vi "Untitled 1 (SubVI).vi"(11 "Path":path) -> (3 "new picture":picture)   [LabVIEW 2020]
panel:
  # "Ceballos Conde Emanuel"
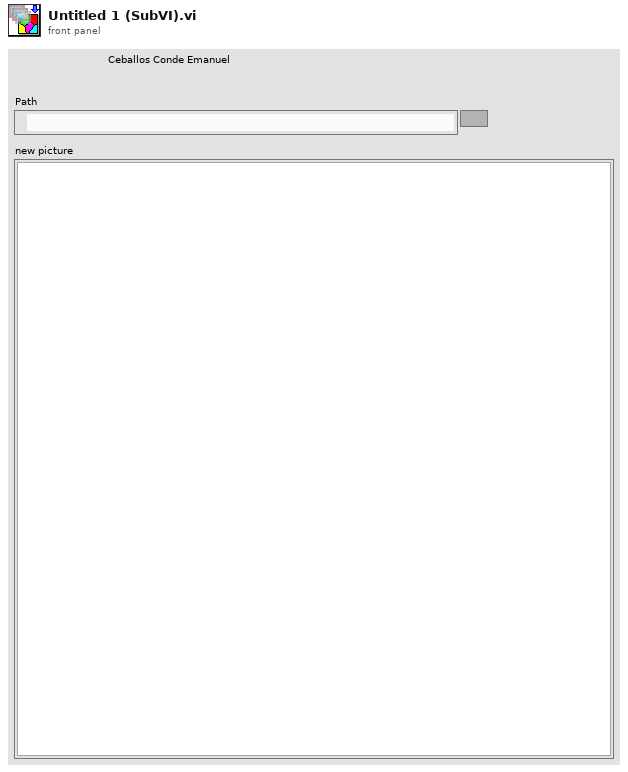
[diagram p1: front panel]
types:
  T1 = enum16{"E1", "E2", "E3", "E4", "E5", "E6", "E7", "E8", "E9"}
  T2 = typedef "imagedata.ctl" = cluster{"image type":i32, "image depth":i32, "image":u8[], "mask":u8[], "colors":u32[], "Rectangle":cluster{"left":i16, "top":i16, "right":i16, "bottom":i16}}
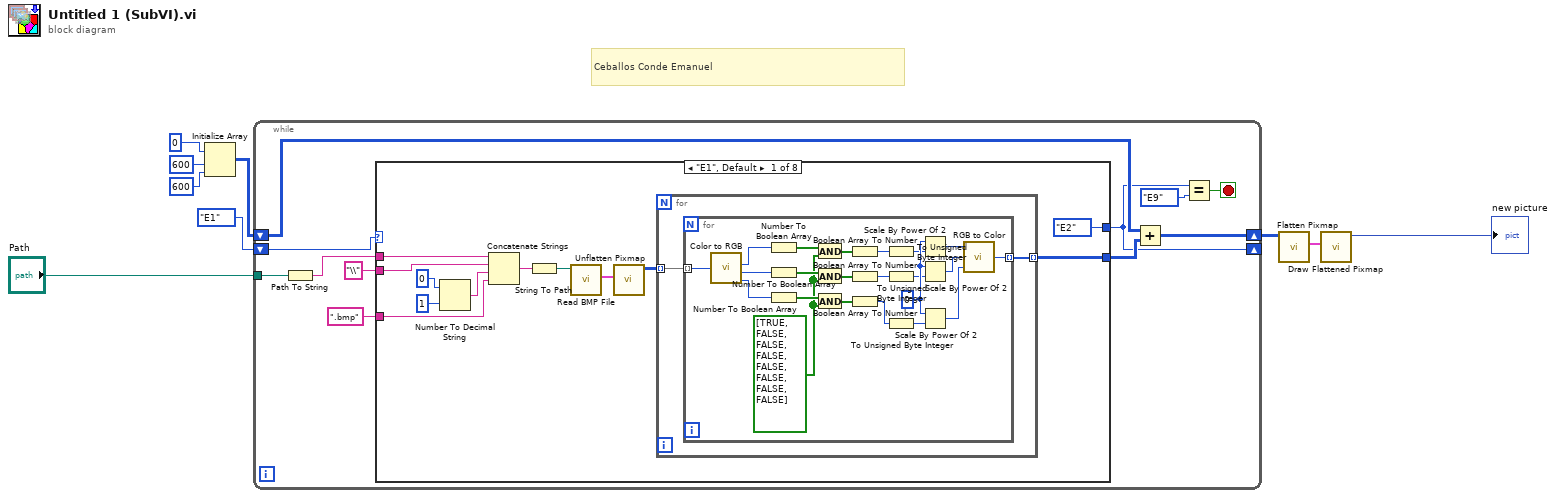
[diagram p0: block diagram]
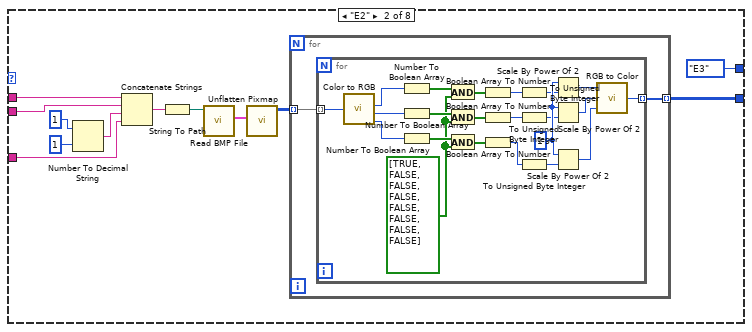
[diagram p2: hidden frame]
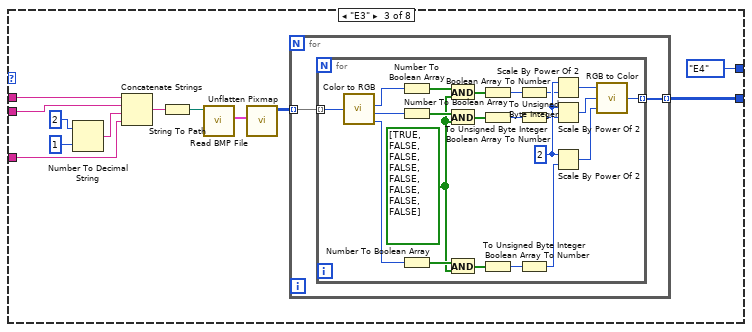
[diagram p3: hidden frame]
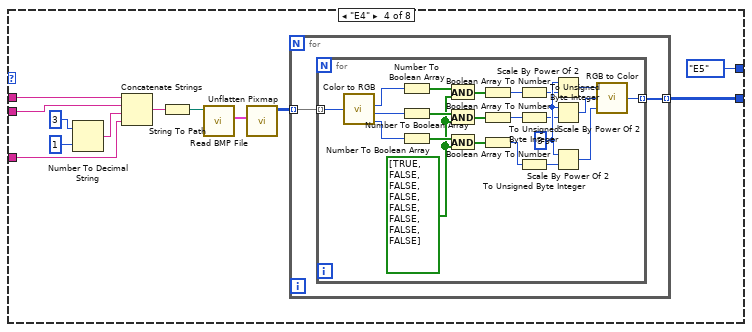
[diagram p4: hidden frame]
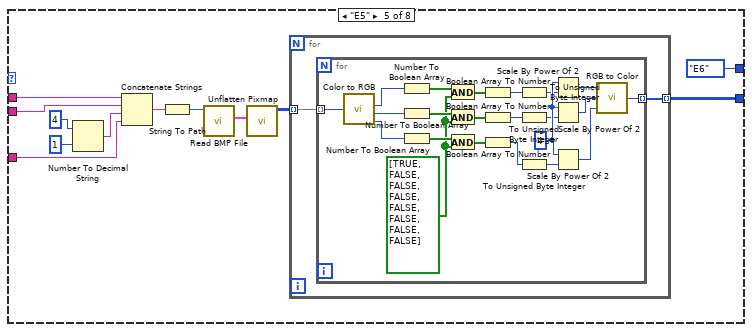
[diagram p5: hidden frame]
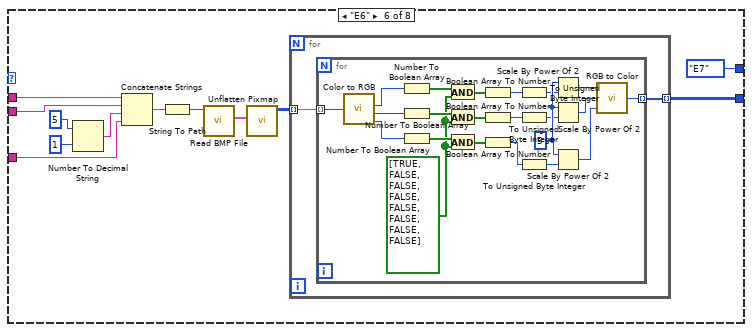
[diagram p6: hidden frame]
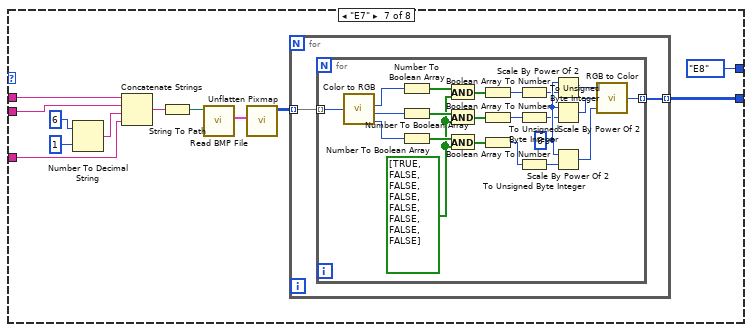
[diagram p7: hidden frame]
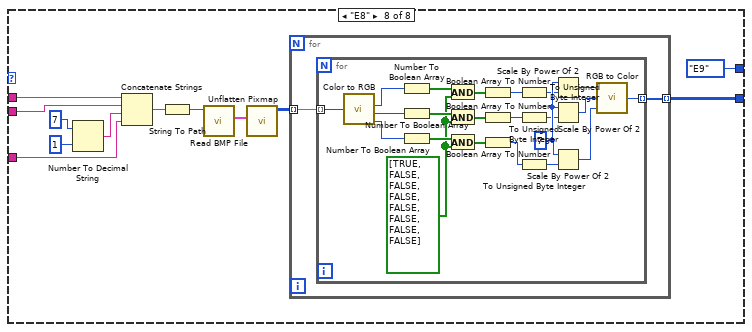
[diagram p8: hidden frame]
diagram:
  # "Ceballos Conde Emanuel"
  n1 = Initialize Array(u32 0 ("element"), 600 ("dimension size"), 600 ("dimension size")) -> (w5:u32[][])
  n2 = while {
    shift-right: [w15] -> _
    shift-left: T1."E1" -> [w20]
    shift-right: [w18] -> w4
    shift-left: w5 -> [w17]
    tunnel: "Path" -> [w10]
    stop <- w16 stop-if-true
    n3 = Path To String(path=w10) -> (string=w13:string)
    n4 = case shown="\"E1\", Default" w20 {
      tunnel: [w31 w66 w102 w138 w174 w210 w246 w282] -> w19
      tunnel: [T1."E2" T1."E3" T1."E4" T1."E5" T1."E6" T1."E7" T1."E8" T1."E9"] -> w15
      tunnel: w13 -> [w28 w60 w94 w130 w168 w205 w240 w276]
      tunnel: "\\" ("string") -> [w27 w59 w93 w129 w167 w204 w239 w275]
      tunnel: ".bmp" -> [w23 w57 w96 w132 w165 w203 w237 w273]
      frame "E1", Default {
        n5 = Number To Decimal String(number=0, width (-)=i16 1) -> (decimal integer string=w26:string)
        n6 = Concatenate Strings(w28, w27, w26, w23) -> (w21:string)
        n7 = String To Path(string=w21) -> (path=w22:path)
        n8 = call <vilib>:"Read BMP File.vi"("path to BMP file"=w22) -> ("image data"=w30:T2)  [unwired: 8 in, 2 out]
        n9 = call <vilib>:"Unflatten Pixmap.vi"("image data"=w30) -> ("24-bit pixmap"=w32:u32[][])  [unwired: 4 in, 6 out]
        n10 = for {
          tunnel: w32 -> [w34] mode=indexing
          tunnel: [w33] -> w31 mode=indexing
          n11 = for {
            tunnel: w34 -> [w56] mode=indexing
            tunnel: [w39] -> w33 mode=indexing
            w35 = bool[] [TRUE, FALSE, FALSE, FALSE, FALSE, FALSE, FALSE, FALSE] ("Boolean array 7")
            w42 = u8 0 ("x")
            n12 = call <vilib>:"Color to RGB.vi"("Color"=w56) -> ("R"=w53:u8, "G"=w48:u8, "B"=w47:u8)  [unwired: 1 out]
            n13 = Number To Boolean Array(number=w53) -> (Boolean array=w55:bool[])
            n14 = Number To Boolean Array(number=w48) -> (Boolean array=w52:bool[])
            n15 = Number To Boolean Array(number=w47) -> (Boolean array=w50:bool[])
            n16 = And(x=w55, y=w35) -> (x .and. y?=w54:bool[])
            n17 = And(x=w52, y=w35) -> (x .and. y?=w51:bool[])
            n18 = And(x=w50, y=w35) -> (x .and. y?=w49:bool[])
            n19 = Boolean Array To Number(Boolean array=w54) -> (number=w43:u32)
            n20 = Boolean Array To Number(Boolean array=w51) -> (number=w40:u32)
            n21 = Boolean Array To Number(Boolean array=w49) -> (number=w41:u32)
            n22 = To Unsigned Byte Integer(number=w43) -> (unsigned 8bit integer=w38:u8)
            n23 = To Unsigned Byte Integer(number=w40) -> (unsigned 8bit integer=w37:u8)
            n24 = To Unsigned Byte Integer(number=w41) -> (unsigned 8bit integer=w36:u8)
            n25 = Scale By Power Of 2(n=w42, x=w38) -> (x*2^n=w46:u8)
            n26 = Scale By Power Of 2(n=w42, x=w37) -> (x*2^n=w45:u8)
            n27 = Scale By Power Of 2(n=w42, x=w36) -> (x*2^n=w44:u8)
            n28 = call <vilib>:"RGB to Color.vi"("B"=w44, "G"=w45, "R"=w46) -> ("Color"=w39:u32)
          }
        }
      }
      frame "E2" {
        n29 = Number To Decimal String(number=1, width (-)=i16 1) -> (decimal integer string=w58:string)
        n30 = Concatenate Strings(w60, w59, w58, w57) -> (w64:string)
        n31 = String To Path(string=w64) -> (path=w61:path)
        n32 = call <vilib>:"Read BMP File.vi"("path to BMP file"=w61) -> ("image data"=w68:T2)  [unwired: 8 in, 2 out]
        n33 = call <vilib>:"Unflatten Pixmap.vi"("image data"=w68) -> ("24-bit pixmap"=w67:u32[][])  [unwired: 4 in, 6 out]
        n34 = for {
          tunnel: w67 -> [w70] mode=indexing
          tunnel: [w69] -> w66 mode=indexing
          n35 = for {
            tunnel: w70 -> [w92] mode=indexing
            tunnel: [w75] -> w69 mode=indexing
            w71 = bool[] [TRUE, FALSE, FALSE, FALSE, FALSE, FALSE, FALSE, FALSE] ("Boolean array 7")
            w78 = u8 1 ("x")
            n36 = call <vilib>:"Color to RGB.vi"("Color"=w92) -> ("R"=w89:u8, "G"=w84:u8, "B"=w83:u8)  [unwired: 1 out]
            n37 = Number To Boolean Array(number=w89) -> (Boolean array=w91:bool[])
            n38 = Number To Boolean Array(number=w84) -> (Boolean array=w88:bool[])
            n39 = Number To Boolean Array(number=w83) -> (Boolean array=w86:bool[])
            n40 = And(x=w91, y=w71) -> (x .and. y?=w90:bool[])
            n41 = And(x=w88, y=w71) -> (x .and. y?=w87:bool[])
            n42 = And(x=w86, y=w71) -> (x .and. y?=w85:bool[])
            n43 = Boolean Array To Number(Boolean array=w90) -> (number=w79:u32)
            n44 = Boolean Array To Number(Boolean array=w87) -> (number=w76:u32)
            n45 = Boolean Array To Number(Boolean array=w85) -> (number=w77:u32)
            n46 = To Unsigned Byte Integer(number=w79) -> (unsigned 8bit integer=w74:u8)
            n47 = To Unsigned Byte Integer(number=w76) -> (unsigned 8bit integer=w73:u8)
            n48 = To Unsigned Byte Integer(number=w77) -> (unsigned 8bit integer=w72:u8)
            n49 = Scale By Power Of 2(n=w78, x=w74) -> (x*2^n=w82:u8)
            n50 = Scale By Power Of 2(n=w78, x=w73) -> (x*2^n=w81:u8)
            n51 = Scale By Power Of 2(n=w78, x=w72) -> (x*2^n=w80:u8)
            n52 = call <vilib>:"RGB to Color.vi"("B"=w80, "G"=w81, "R"=w82) -> ("Color"=w75:u32)
          }
        }
      }
      frame "E3" {
        n53 = Number To Decimal String(number=2, width (-)=i16 1) -> (decimal integer string=w95:string)
        n54 = Concatenate Strings(w94, w93, w95, w96) -> (w100:string)
        n55 = String To Path(string=w100) -> (path=w97:path)
        n56 = call <vilib>:"Read BMP File.vi"("path to BMP file"=w97) -> ("image data"=w104:T2)  [unwired: 8 in, 2 out]
        n57 = call <vilib>:"Unflatten Pixmap.vi"("image data"=w104) -> ("24-bit pixmap"=w103:u32[][])  [unwired: 4 in, 6 out]
        n58 = for {
          tunnel: w103 -> [w106] mode=indexing
          tunnel: [w105] -> w102 mode=indexing
          n59 = for {
            tunnel: w106 -> [w128] mode=indexing
            tunnel: [w111] -> w105 mode=indexing
            w107 = bool[] [TRUE, FALSE, FALSE, FALSE, FALSE, FALSE, FALSE, FALSE] ("Boolean array 7")
            w114 = u8 2 ("x")
            n60 = call <vilib>:"Color to RGB.vi"("Color"=w128) -> ("R"=w125:u8, "G"=w120:u8, "B"=w119:u8)  [unwired: 1 out]
            n61 = Number To Boolean Array(number=w125) -> (Boolean array=w127:bool[])
            n62 = Number To Boolean Array(number=w120) -> (Boolean array=w124:bool[])
            n63 = Number To Boolean Array(number=w119) -> (Boolean array=w122:bool[])
            n64 = And(x=w127, y=w107) -> (x .and. y?=w126:bool[])
            n65 = And(x=w124, y=w107) -> (x .and. y?=w123:bool[])
            n66 = And(x=w122, y=w107) -> (x .and. y?=w121:bool[])
            n67 = Boolean Array To Number(Boolean array=w126) -> (number=w115:u32)
            n68 = Boolean Array To Number(Boolean array=w123) -> (number=w112:u32)
            n69 = Boolean Array To Number(Boolean array=w121) -> (number=w113:u32)
            n70 = To Unsigned Byte Integer(number=w115) -> (unsigned 8bit integer=w110:u8)
            n71 = To Unsigned Byte Integer(number=w112) -> (unsigned 8bit integer=w109:u8)
            n72 = To Unsigned Byte Integer(number=w113) -> (unsigned 8bit integer=w108:u8)
            n73 = Scale By Power Of 2(n=w114, x=w110) -> (x*2^n=w118:u8)
            n74 = Scale By Power Of 2(n=w114, x=w109) -> (x*2^n=w117:u8)
            n75 = Scale By Power Of 2(n=w114, x=w108) -> (x*2^n=w116:u8)
            n76 = call <vilib>:"RGB to Color.vi"("B"=w116, "G"=w117, "R"=w118) -> ("Color"=w111:u32)
          }
        }
      }
      frame "E4" {
        n77 = Number To Decimal String(number=3, width (-)=i16 1) -> (decimal integer string=w131:string)
        n78 = Concatenate Strings(w130, w129, w131, w132) -> (w136:string)
        n79 = String To Path(string=w136) -> (path=w133:path)
        n80 = call <vilib>:"Read BMP File.vi"("path to BMP file"=w133) -> ("image data"=w140:T2)  [unwired: 8 in, 2 out]
        n81 = call <vilib>:"Unflatten Pixmap.vi"("image data"=w140) -> ("24-bit pixmap"=w139:u32[][])  [unwired: 4 in, 6 out]
        n82 = for {
          tunnel: w139 -> [w142] mode=indexing
          tunnel: [w141] -> w138 mode=indexing
          n83 = for {
            tunnel: w142 -> [w164] mode=indexing
            tunnel: [w147] -> w141 mode=indexing
            w143 = bool[] [TRUE, FALSE, FALSE, FALSE, FALSE, FALSE, FALSE, FALSE] ("Boolean array 7")
            w150 = u8 3 ("x")
            n84 = call <vilib>:"Color to RGB.vi"("Color"=w164) -> ("R"=w161:u8, "G"=w156:u8, "B"=w155:u8)  [unwired: 1 out]
            n85 = Number To Boolean Array(number=w161) -> (Boolean array=w163:bool[])
            n86 = Number To Boolean Array(number=w156) -> (Boolean array=w160:bool[])
            n87 = Number To Boolean Array(number=w155) -> (Boolean array=w158:bool[])
            n88 = And(x=w163, y=w143) -> (x .and. y?=w162:bool[])
            n89 = And(x=w160, y=w143) -> (x .and. y?=w159:bool[])
            n90 = And(x=w158, y=w143) -> (x .and. y?=w157:bool[])
            n91 = Boolean Array To Number(Boolean array=w162) -> (number=w151:u32)
            n92 = Boolean Array To Number(Boolean array=w159) -> (number=w148:u32)
            n93 = Boolean Array To Number(Boolean array=w157) -> (number=w149:u32)
            n94 = To Unsigned Byte Integer(number=w151) -> (unsigned 8bit integer=w146:u8)
            n95 = To Unsigned Byte Integer(number=w148) -> (unsigned 8bit integer=w145:u8)
            n96 = To Unsigned Byte Integer(number=w149) -> (unsigned 8bit integer=w144:u8)
            n97 = Scale By Power Of 2(n=w150, x=w146) -> (x*2^n=w154:u8)
            n98 = Scale By Power Of 2(n=w150, x=w145) -> (x*2^n=w153:u8)
            n99 = Scale By Power Of 2(n=w150, x=w144) -> (x*2^n=w152:u8)
            n100 = call <vilib>:"RGB to Color.vi"("B"=w152, "G"=w153, "R"=w154) -> ("Color"=w147:u32)
          }
        }
      }
      frame "E5" {
        n101 = Number To Decimal String(number=4, width (-)=i16 1) -> (decimal integer string=w166:string)
        n102 = Concatenate Strings(w168, w167, w166, w165) -> (w170:string)
        n103 = String To Path(string=w170) -> (path=w169:path)
        n104 = call <vilib>:"Read BMP File.vi"("path to BMP file"=w169) -> ("image data"=w176:T2)  [unwired: 8 in, 2 out]
        n105 = call <vilib>:"Unflatten Pixmap.vi"("image data"=w176) -> ("24-bit pixmap"=w175:u32[][])  [unwired: 4 in, 6 out]
        n106 = for {
          tunnel: w175 -> [w178] mode=indexing
          tunnel: [w177] -> w174 mode=indexing
          n107 = for {
            tunnel: w178 -> [w200] mode=indexing
            tunnel: [w183] -> w177 mode=indexing
            w179 = bool[] [TRUE, FALSE, FALSE, FALSE, FALSE, FALSE, FALSE, FALSE] ("Boolean array 7")
            w186 = u8 4 ("x")
            n108 = call <vilib>:"Color to RGB.vi"("Color"=w200) -> ("R"=w197:u8, "G"=w192:u8, "B"=w191:u8)  [unwired: 1 out]
            n109 = Number To Boolean Array(number=w197) -> (Boolean array=w199:bool[])
            n110 = Number To Boolean Array(number=w192) -> (Boolean array=w196:bool[])
            n111 = Number To Boolean Array(number=w191) -> (Boolean array=w194:bool[])
            n112 = And(x=w199, y=w179) -> (x .and. y?=w198:bool[])
            n113 = And(x=w196, y=w179) -> (x .and. y?=w195:bool[])
            n114 = And(x=w194, y=w179) -> (x .and. y?=w193:bool[])
            n115 = Boolean Array To Number(Boolean array=w198) -> (number=w187:u32)
            n116 = Boolean Array To Number(Boolean array=w195) -> (number=w184:u32)
            n117 = Boolean Array To Number(Boolean array=w193) -> (number=w185:u32)
            n118 = To Unsigned Byte Integer(number=w187) -> (unsigned 8bit integer=w182:u8)
            n119 = To Unsigned Byte Integer(number=w184) -> (unsigned 8bit integer=w181:u8)
            n120 = To Unsigned Byte Integer(number=w185) -> (unsigned 8bit integer=w180:u8)
            n121 = Scale By Power Of 2(n=w186, x=w182) -> (x*2^n=w190:u8)
            n122 = Scale By Power Of 2(n=w186, x=w181) -> (x*2^n=w189:u8)
            n123 = Scale By Power Of 2(n=w186, x=w180) -> (x*2^n=w188:u8)
            n124 = call <vilib>:"RGB to Color.vi"("B"=w188, "G"=w189, "R"=w190) -> ("Color"=w183:u32)
          }
        }
      }
      frame "E6" {
        n125 = Number To Decimal String(number=5, width (-)=i16 1) -> (decimal integer string=w202:string)
        n126 = Concatenate Strings(w205, w204, w202, w203) -> (w206:string)
        n127 = String To Path(string=w206) -> (path=w201:path)
        n128 = call <vilib>:"Read BMP File.vi"("path to BMP file"=w201) -> ("image data"=w212:T2)  [unwired: 8 in, 2 out]
        n129 = call <vilib>:"Unflatten Pixmap.vi"("image data"=w212) -> ("24-bit pixmap"=w211:u32[][])  [unwired: 4 in, 6 out]
        n130 = for {
          tunnel: w211 -> [w214] mode=indexing
          tunnel: [w213] -> w210 mode=indexing
          n131 = for {
            tunnel: w214 -> [w236] mode=indexing
            tunnel: [w219] -> w213 mode=indexing
            w215 = bool[] [TRUE, FALSE, FALSE, FALSE, FALSE, FALSE, FALSE, FALSE] ("Boolean array 7")
            w222 = u8 5 ("x")
            n132 = call <vilib>:"Color to RGB.vi"("Color"=w236) -> ("R"=w233:u8, "G"=w228:u8, "B"=w227:u8)  [unwired: 1 out]
            n133 = Number To Boolean Array(number=w233) -> (Boolean array=w235:bool[])
            n134 = Number To Boolean Array(number=w228) -> (Boolean array=w232:bool[])
            n135 = Number To Boolean Array(number=w227) -> (Boolean array=w230:bool[])
            n136 = And(x=w235, y=w215) -> (x .and. y?=w234:bool[])
            n137 = And(x=w232, y=w215) -> (x .and. y?=w231:bool[])
            n138 = And(x=w230, y=w215) -> (x .and. y?=w229:bool[])
            n139 = Boolean Array To Number(Boolean array=w234) -> (number=w223:u32)
            n140 = Boolean Array To Number(Boolean array=w231) -> (number=w220:u32)
            n141 = Boolean Array To Number(Boolean array=w229) -> (number=w221:u32)
            n142 = To Unsigned Byte Integer(number=w223) -> (unsigned 8bit integer=w218:u8)
            n143 = To Unsigned Byte Integer(number=w220) -> (unsigned 8bit integer=w217:u8)
            n144 = To Unsigned Byte Integer(number=w221) -> (unsigned 8bit integer=w216:u8)
            n145 = Scale By Power Of 2(n=w222, x=w218) -> (x*2^n=w226:u8)
            n146 = Scale By Power Of 2(n=w222, x=w217) -> (x*2^n=w225:u8)
            n147 = Scale By Power Of 2(n=w222, x=w216) -> (x*2^n=w224:u8)
            n148 = call <vilib>:"RGB to Color.vi"("B"=w224, "G"=w225, "R"=w226) -> ("Color"=w219:u32)
          }
        }
      }
      frame "E7" {
        n149 = Number To Decimal String(number=6, width (-)=i16 1) -> (decimal integer string=w238:string)
        n150 = Concatenate Strings(w240, w239, w238, w237) -> (w242:string)
        n151 = String To Path(string=w242) -> (path=w241:path)
        n152 = call <vilib>:"Read BMP File.vi"("path to BMP file"=w241) -> ("image data"=w248:T2)  [unwired: 8 in, 2 out]
        n153 = call <vilib>:"Unflatten Pixmap.vi"("image data"=w248) -> ("24-bit pixmap"=w247:u32[][])  [unwired: 4 in, 6 out]
        n154 = for {
          tunnel: w247 -> [w250] mode=indexing
          tunnel: [w249] -> w246 mode=indexing
          n155 = for {
            tunnel: w250 -> [w272] mode=indexing
            tunnel: [w255] -> w249 mode=indexing
            w251 = bool[] [TRUE, FALSE, FALSE, FALSE, FALSE, FALSE, FALSE, FALSE] ("Boolean array 7")
            w258 = u8 6 ("x")
            n156 = call <vilib>:"Color to RGB.vi"("Color"=w272) -> ("R"=w269:u8, "G"=w264:u8, "B"=w263:u8)  [unwired: 1 out]
            n157 = Number To Boolean Array(number=w269) -> (Boolean array=w271:bool[])
            n158 = Number To Boolean Array(number=w264) -> (Boolean array=w268:bool[])
            n159 = Number To Boolean Array(number=w263) -> (Boolean array=w266:bool[])
            n160 = And(x=w271, y=w251) -> (x .and. y?=w270:bool[])
            n161 = And(x=w268, y=w251) -> (x .and. y?=w267:bool[])
            n162 = And(x=w266, y=w251) -> (x .and. y?=w265:bool[])
            n163 = Boolean Array To Number(Boolean array=w270) -> (number=w259:u32)
            n164 = Boolean Array To Number(Boolean array=w267) -> (number=w256:u32)
            n165 = Boolean Array To Number(Boolean array=w265) -> (number=w257:u32)
            n166 = To Unsigned Byte Integer(number=w259) -> (unsigned 8bit integer=w254:u8)
            n167 = To Unsigned Byte Integer(number=w256) -> (unsigned 8bit integer=w253:u8)
            n168 = To Unsigned Byte Integer(number=w257) -> (unsigned 8bit integer=w252:u8)
            n169 = Scale By Power Of 2(n=w258, x=w254) -> (x*2^n=w262:u8)
            n170 = Scale By Power Of 2(n=w258, x=w253) -> (x*2^n=w261:u8)
            n171 = Scale By Power Of 2(n=w258, x=w252) -> (x*2^n=w260:u8)
            n172 = call <vilib>:"RGB to Color.vi"("B"=w260, "G"=w261, "R"=w262) -> ("Color"=w255:u32)
          }
        }
      }
      frame "E8" {
        n173 = Number To Decimal String(number=7, width (-)=i16 1) -> (decimal integer string=w274:string)
        n174 = Concatenate Strings(w276, w275, w274, w273) -> (w278:string)
        n175 = String To Path(string=w278) -> (path=w277:path)
        n176 = call <vilib>:"Read BMP File.vi"("path to BMP file"=w277) -> ("image data"=w283:T2)  [unwired: 8 in, 2 out]
        n177 = call <vilib>:"Unflatten Pixmap.vi"("image data"=w283) -> ("24-bit pixmap"=w284:u32[][])  [unwired: 4 in, 6 out]
        n178 = for {
          tunnel: w284 -> [w286] mode=indexing
          tunnel: [w285] -> w282 mode=indexing
          n179 = for {
            tunnel: w286 -> [w308] mode=indexing
            tunnel: [w291] -> w285 mode=indexing
            w287 = bool[] [TRUE, FALSE, FALSE, FALSE, FALSE, FALSE, FALSE, FALSE] ("Boolean array 7")
            w294 = u8 7 ("x")
            n180 = call <vilib>:"Color to RGB.vi"("Color"=w308) -> ("R"=w305:u8, "G"=w300:u8, "B"=w299:u8)  [unwired: 1 out]
            n181 = Number To Boolean Array(number=w305) -> (Boolean array=w307:bool[])
            n182 = Number To Boolean Array(number=w300) -> (Boolean array=w304:bool[])
            n183 = Number To Boolean Array(number=w299) -> (Boolean array=w302:bool[])
            n184 = And(x=w307, y=w287) -> (x .and. y?=w306:bool[])
            n185 = And(x=w304, y=w287) -> (x .and. y?=w303:bool[])
            n186 = And(x=w302, y=w287) -> (x .and. y?=w301:bool[])
            n187 = Boolean Array To Number(Boolean array=w306) -> (number=w295:u32)
            n188 = Boolean Array To Number(Boolean array=w303) -> (number=w292:u32)
            n189 = Boolean Array To Number(Boolean array=w301) -> (number=w293:u32)
            n190 = To Unsigned Byte Integer(number=w295) -> (unsigned 8bit integer=w290:u8)
            n191 = To Unsigned Byte Integer(number=w292) -> (unsigned 8bit integer=w289:u8)
            n192 = To Unsigned Byte Integer(number=w293) -> (unsigned 8bit integer=w288:u8)
            n193 = Scale By Power Of 2(n=w294, x=w290) -> (x*2^n=w298:u8)
            n194 = Scale By Power Of 2(n=w294, x=w289) -> (x*2^n=w297:u8)
            n195 = Scale By Power Of 2(n=w294, x=w288) -> (x*2^n=w296:u8)
            n196 = call <vilib>:"RGB to Color.vi"("B"=w296, "G"=w297, "R"=w298) -> ("Color"=w291:u32)
          }
        }
      }
    }
    n197 = Add(x=w17, y=w19) -> (x+y=w18:u32[][])
    n198 = Equal?(x=w15, y=T1."E9") -> (x = y?=w16:bool)
  }
  n199 = call <vilib>:"Flatten Pixmap.vi"("24-bit pixmap"=w4) -> ("image data"=w2:T2)  [unwired: 10 in]
  n200 = call <vilib>:"Draw Flattened Pixmap.vi"("image data"=w2) -> ("new picture"=→"new picture":picture)  [unwired: 8 in]
